vi "libtiff3_write_tiff page SGL.vi"(0 "Handle":i32, 1 "Image Pixels (Float)":sgl[][](array[numeric]) format="%.2f", 4 "Image Description":string, 5 "error in (no error)":errorcluster, 6 "page":u32, 7 "x.pixels":i32, 8 "totalpages":i32, 9 "y.pixels":i32) -> (14 "Handle out":i32, 19 "error out":errorcluster)   [LabVIEW 2020]
doc: "SciScan 1.0 151216\nWrite a SGL (32-bit IEEE) page using LIBTIFFwriteScanLine to a file previously open for writing"
uses:
  DLLs/libtiff3 (32).dll
panel:
  out "status_sampleformat":i32
  out "status_compression":i32
  out "status width":i32
  out "status_length":i32
  out "status_spp":i32
  out "status_bps":i32
  out "status_orientation":i32
  out "status_planarconfig":i32
  out "status_photo":i32
  out "status_writscanline":i32
  out "status_subfile":i32
  out "status_writedir":i32
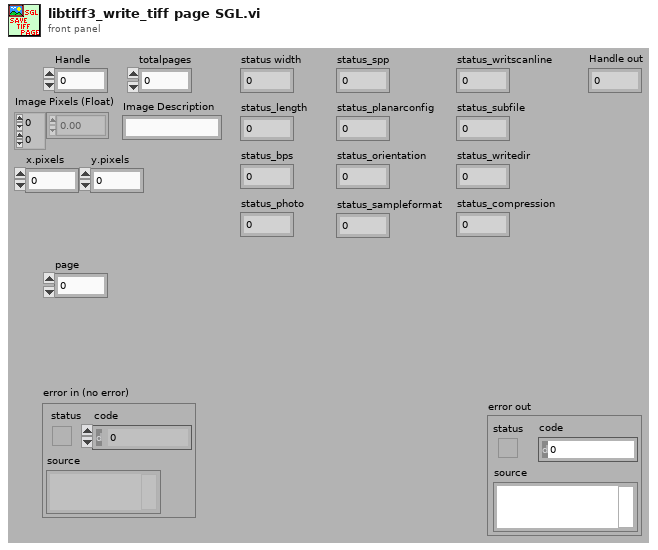
[diagram p1: front panel]
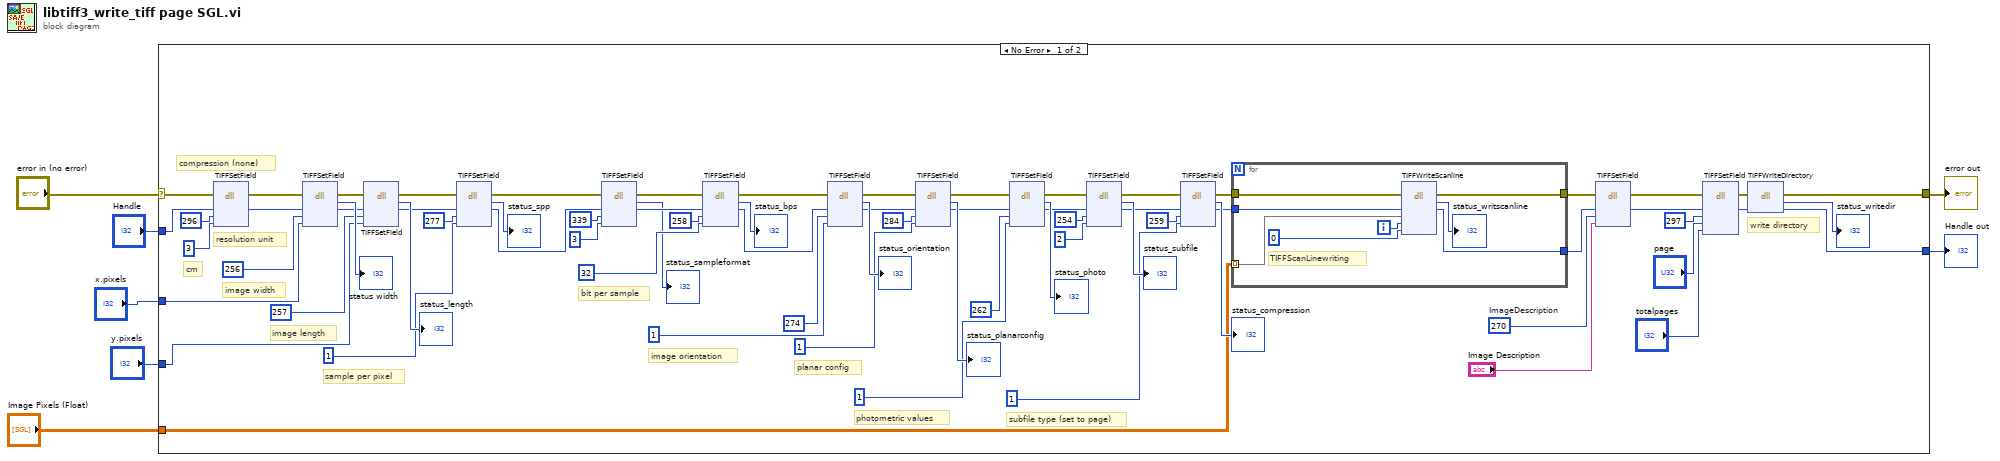
[diagram p0: block diagram]
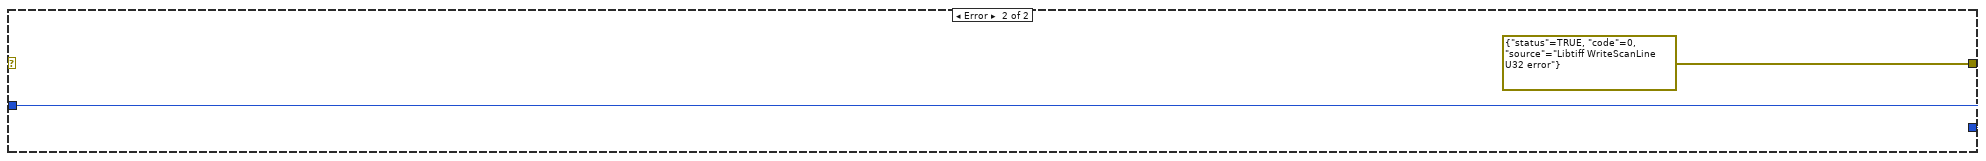
[diagram p2: hidden frame]
diagram:
  n1 = case shown="No Error" "error in (no error)" {
    selector: "error in (no error)" -> [w18 _]
    tunnel: "Handle" -> [w19 w88]
    tunnel: [w50 w88] -> w1
    tunnel: [w38 errorcluster {"status"=TRUE, "code"=0, "source"="Libtiff WriteScanLine U32 error"} ("error out")] -> w6
    tunnel: "Image Pixels (Float)" -> [w24 _]
    tunnel: "x.pixels" -> [w23 _]
    tunnel: "y.pixels" -> [w22 _]
    frame No Error {
      w10 = 270  # ImageDescription
      # "cm"
      # "resolution unit"
      # "compression (none)"
      # "write directory"
      # "subfile type (set to page)"
      # "photometric values"
      # "planar config"
      # "image orientation"
      # "bit per sample"
      # "sample per pixel"
      # "image length"
      # "image width"
      n2 = dll-call lib="C:/LocalSVNSCC/Microscope-Software-Commonised-LV/branches/release_3.2_stable_lv2020/support/Libtiff3/DLLs/libtiff3 (32).dll" fn="TIFFSetField"(error in=w18, "Handle"=w19, "TIFF_tag"=296, "value"=u32 3) -> (error out=w17:errorcluster, "Handle"=w16:i32)  [unwired: 4 in, 2 out]
      n3 = dll-call lib="C:/LocalSVNSCC/Microscope-Software-Commonised-LV/branches/release_3.2_stable_lv2020/support/Libtiff3/DLLs/libtiff3 (32).dll" fn="TIFFSetField"(error in=w17, "Handle"=w16, "TIFF_tag"=256, "Value"=w23) -> (error out=w45:errorcluster, "return type"=→"status width":i32, "Handle"=w76:i32)  [unwired: 4 in, 1 out]
      n4 = dll-call lib="C:/LocalSVNSCC/Microscope-Software-Commonised-LV/branches/release_3.2_stable_lv2020/support/Libtiff3/DLLs/libtiff3 (32).dll" fn="TIFFSetField"(error in=w45, "Handle"=w76, "TIFF_tag"=257, "value"=w22) -> (error out=w44:errorcluster, "return type"=→"status_length":i32, "Handle"=w73:i32)  [unwired: 4 in, 1 out]
      n5 = dll-call lib="C:/LocalSVNSCC/Microscope-Software-Commonised-LV/branches/release_3.2_stable_lv2020/support/Libtiff3/DLLs/libtiff3 (32).dll" fn="TIFFSetField"(error in=w44, "Handle"=w73, "TIFF_tag"=277, "value"=u32 1) -> (error out=w27:errorcluster, "return type"=→"status_spp":i32, "Handle"=w31:i32)  [unwired: 4 in, 1 out]
      n6 = dll-call lib="C:/LocalSVNSCC/Microscope-Software-Commonised-LV/branches/release_3.2_stable_lv2020/support/Libtiff3/DLLs/libtiff3 (32).dll" fn="TIFFSetField"(error in=w27, "Handle"=w31, "TIFF_tag"=339, "value"=u32 3) -> (error out=w26:errorcluster, "return type"=→"status_sampleformat":i32, "Handle"=w28:i32)  [unwired: 4 in, 1 out]
      n7 = dll-call lib="C:/LocalSVNSCC/Microscope-Software-Commonised-LV/branches/release_3.2_stable_lv2020/support/Libtiff3/DLLs/libtiff3 (32).dll" fn="TIFFSetField"(error in=w26, "Handle"=w28, "TIFF_tag"=258, "value"=u32 32) -> (error out=w43:errorcluster, "return type"=→"status_bps":i32, "Handle"=w68:i32)  [unwired: 4 in, 1 out]
      n8 = dll-call lib="C:/LocalSVNSCC/Microscope-Software-Commonised-LV/branches/release_3.2_stable_lv2020/support/Libtiff3/DLLs/libtiff3 (32).dll" fn="TIFFSetField"(error in=w43, "Handle"=w68, "TIFF_tag"=274, "value"=u32 1) -> (error out=w42:errorcluster, "return type"=→"status_orientation":i32, "Handle"=w64:i32)  [unwired: 4 in, 1 out]
      n9 = dll-call lib="C:/LocalSVNSCC/Microscope-Software-Commonised-LV/branches/release_3.2_stable_lv2020/support/Libtiff3/DLLs/libtiff3 (32).dll" fn="TIFFSetField"(error in=w42, "Handle"=w64, "TIFF_tag"=284, "value"=u32 1) -> (error out=w41:errorcluster, "return type"=→"status_planarconfig":i32, "Handle"=w60:i32)  [unwired: 4 in, 1 out]
      n10 = dll-call lib="C:/LocalSVNSCC/Microscope-Software-Commonised-LV/branches/release_3.2_stable_lv2020/support/Libtiff3/DLLs/libtiff3 (32).dll" fn="TIFFSetField"(error in=w41, "Handle"=w60, "TIFF_tag"=262, "value"=u32 1) -> (error out=w40:errorcluster, "return type"=→"status_photo":i32, "Handle"=w55:i32)  [unwired: 4 in, 1 out]
      n11 = dll-call lib="C:/LocalSVNSCC/Microscope-Software-Commonised-LV/branches/release_3.2_stable_lv2020/support/Libtiff3/DLLs/libtiff3 (32).dll" fn="TIFFSetField"(error in=w40, "Handle"=w55, "TIFF_tag"=254, "value"=u32 2) -> (error out=w39:errorcluster, "return type"=→"status_subfile":i32, "Handle"=w47:i32)  [unwired: 4 in, 1 out]
      n12 = dll-call lib="C:/LocalSVNSCC/Microscope-Software-Commonised-LV/branches/release_3.2_stable_lv2020/support/Libtiff3/DLLs/libtiff3 (32).dll" fn="TIFFSetField"(error in=w39, "Handle"=w47, "TIFF_tag"=259, "value"=u32 1) -> (error out=w15:errorcluster, "return type"=→"status_compression":i32, "Handle"=w14:i32)  [unwired: 4 in, 1 out]
      n13 = for {
        tunnel: [w85] -> w8
        tunnel: [w84] -> w9
        tunnel: w14 -> [w82]
        tunnel: w15 -> [w83]
        tunnel: w24 -> [w79] mode=indexing
        i -> [w81]
        # "TIFFScanLinewriting"
        n14 = dll-call lib="C:/LocalSVNSCC/Microscope-Software-Commonised-LV/branches/release_3.2_stable_lv2020/support/Libtiff3/DLLs/libtiff3 (32).dll" fn="TIFFWriteScanline"(error in=w83, "Handle"=w82, "buffer"=w79, "row"=w81, "sample"=0) -> (error out=w84:errorcluster, "return type"=→"status_writscanline":i32, "Handle"=w85:i32)  [unwired: 5 in, 1 out]
      }
      n15 = dll-call lib="C:/LocalSVNSCC/Microscope-Software-Commonised-LV/branches/release_3.2_stable_lv2020/support/Libtiff3/DLLs/libtiff3 (32).dll" fn="TIFFSetField"(error in=w9, "Handle"=w8, "TIFF_tag"=w10, "Value"="Image Description") -> (error out=w13:errorcluster, "Handle"=w12:i32)  [unwired: 4 in, 2 out]
      n16 = dll-call lib="C:/LocalSVNSCC/Microscope-Software-Commonised-LV/branches/release_3.2_stable_lv2020/support/Libtiff3/DLLs/libtiff3 (32).dll" fn="TIFFSetField"(error in=w13, "Handle"=w12, "TIFF_tag"=297, "page"="page", "totalpages"="totalpages") -> (error out=w33:errorcluster, "Handle"=w32:i32)  [unwired: 5 in, 2 out]
      n17 = dll-call lib="C:/LocalSVNSCC/Microscope-Software-Commonised-LV/branches/release_3.2_stable_lv2020/support/Libtiff3/DLLs/libtiff3 (32).dll" fn="TIFFWriteDirectory"(error in=w33, "Handle"=w32) -> (error out=w38:errorcluster, "return type"=→"status_writedir":i32, "Handle"=w50:i32)  [unwired: 2 in, 1 out]
    }
    frame Error {
    }
  }
  "Handle out" <- w1
  "error out" <- w6
